vi "Initialize (SubVI).vi"(8 "error in (no error)":errorcluster, 9 "ID Query (True)":bool=TRUE, 10 "Reset (True)":bool=TRUE, 11 "VISA Refnum in":refnum<visa-resource-name>) -> (0 "error out":errorcluster, 3 "VISA Refnum out":refnum<visa-resource-name>)   [LabVIEW 2023]
uses:
  <vilib>/Instr/_visa.llb/VISA Open Access Mode.ctl
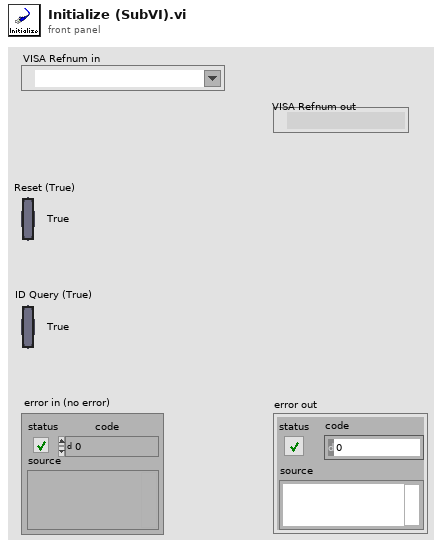
[diagram p1: front panel]
types:
  T1 = typedef "VISA Open Access Mode.ctl" = u32
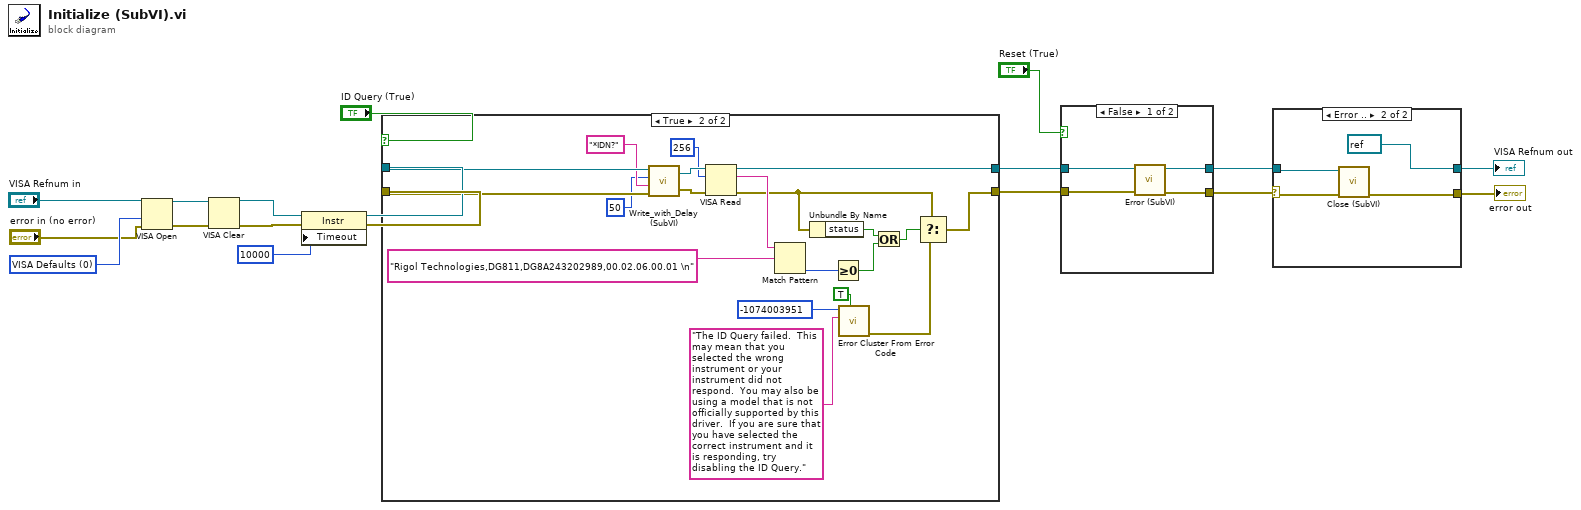
[diagram p0: block diagram]
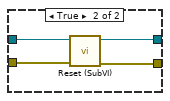
[diagram p3: hidden frame]
diagram:
  w3 = T1 0 items=["VISA Defaults"=0, "Exclusive Lock"=1, "Load Configured Settings"=4] ("Access Mode")
  n1 = VISA Open(access mode=w3, error in (no error)="error in (no error)", VISA resource name="VISA Refnum in") -> (VISA resource name=w4:refnum<visa-resource-name>, error out=w5:errorcluster)  [unwired: 2 in]
  n2 = VISA Clear(VISA resource name=w4, error in (no error)=w5) -> (VISA resource name out=w6:refnum<visa-resource-name>, error out=w7:errorcluster)
  n3 = property class="Instr"(reference=w6, error in=w7, "Timeout"=u32 10000 ("General Settings:Timeout Value")) -> (reference out=w10:refnum<visa-resource-name>, error out=w11:errorcluster)
  n4 = case shown="True" "ID Query (True)" {
    tunnel: w10 -> [w20 w40]
    tunnel: w11 -> [w19 w39]
    tunnel: [w20 w33] -> w13
    tunnel: [w19 w30] -> w14
    frame False {
    }
    frame True {
      n5 = call "Write_with_Delay (SubVI).vi"("error in (no error)"=w39, "Command"="*IDN?", "Delay (500ms)"=50, "VISA Refnum in"=w40) -> ("error out"=w35:errorcluster, "VISA Refnum out"=w36:refnum<visa-resource-name>)
      n6 = VISA Read(VISA resource name=w36, byte count=u32 256, error in (no error)=w35) -> (VISA resource name out=w33:refnum<visa-resource-name>, read buffer=w32:string, error out=w29:errorcluster)  [unwired: 1 out]
      n7 = Match Pattern(string=w32, regular expression="Rigol Technologies,DG811,DG8A243202989,00.02.06.00.01 \n") -> (offset past match=w25:i32)  [unwired: 1 in, 3 out]
      n8 = Unbundle By Name(w29) -> ("status"=w27:bool)
      n9 = Greater Or Equal To 0?(x=w25) -> (x >= 0?=w26:bool)
      n10 = call <vilib>:"Error Cluster From Error Code.vi"("show call chain? (False)"=TRUE, "error message (\"\")"="The ID Query failed.  This may mean that you selected the wrong instrument or your instrument did not respond.  You may also be using a model that is not officially supported by this driver.  If you are sure that you have selected the correct instrument and it is responding, try disabling the ID Query." ("Source (VI Name)"), "error code (0)"=-1074003951 ("Code")) -> ("error out"=w21:errorcluster)  [unwired: 1 in, 5 out]
      n11 = Or(x=w27, y=w26) -> (x .or. y?=w28:bool)
      n12 = Select(t=w29, s=w28, f=w21) -> (s? t:f=w30:errorcluster)
    }
  }
  n13 = case shown="False" "Reset (True)" {
    tunnel: w13 -> [w44 w48]
    tunnel: w14 -> [w43 w47]
    tunnel: [w41 w46] -> w16
    tunnel: [w42 w45] -> w15
    frame False {
      n14 = call "Error (SubVI).vi"("error in (no error)"=w43, "VISA Refnum in"=w44) -> ("error out"=w42:errorcluster, "VISA Refnum out"=w41:refnum<visa-resource-name>)  [unwired: 6 in, 2 out]
    }
    frame True {
      n15 = call "Reset (SubVI).vi"("error in (no error)"=w47, "VISA Refnum in"=w48) -> ("error out"=w45:errorcluster, "VISA Refnum out"=w46:refnum<visa-resource-name>)  [unwired: 8 in]
    }
  }
  n16 = case shown="Error .." w15 {
    selector: w15 -> [w49 w52]
    tunnel: w16 -> [w50 w53]
    tunnel: [w50 refnum<visa-resource-name> refnum ("VISA Refnum out")] -> w17
    tunnel: [w49 w51] -> w18
    frame No Error {
    }
    frame Error {
      n17 = call "Close (SubVI).vi"("error in (no error)"=w52, "VISA Refnum in"=w53) -> ("error out"=w51:errorcluster)  [unwired: 9 in]
    }
  }
  "VISA Refnum out" <- w17
  "error out" <- w18
